vi "ColorArray2Ramp.vi"(11 "Color Array":u32[](array[colorbox])=[0, 16448250, 0]) -> (3 "Color Ramp (zero is black)":u32[](array[colorbox]))   [LabVIEW 2023]
panel:
  # "Overview: This These VI demonstrate algorithms to generate color tables for LabVIEW color ramps.\nRequirements: LabVIEW 2012\nInstructions:\n1. Set colors in color array\n2. Run VI\n3. Change speed\n4. try another colors combination"
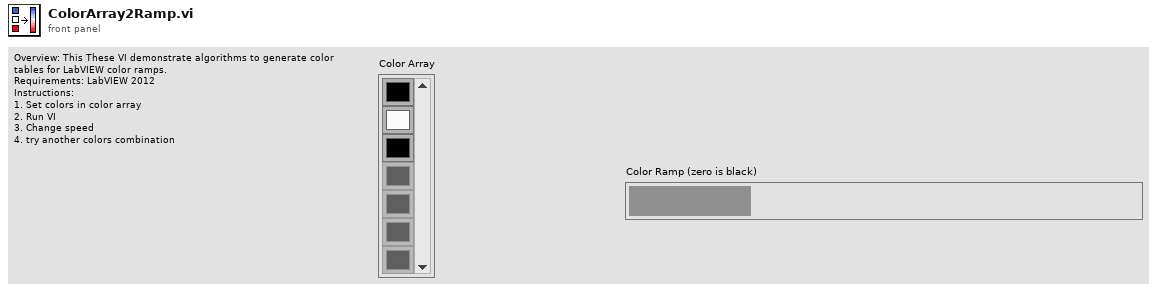
[diagram p1: front panel]
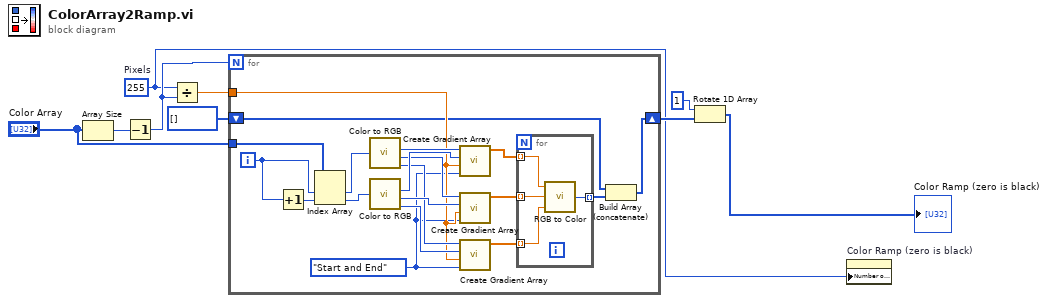
[diagram p0: block diagram]
diagram:
  w1 = 255  # Pixels
  n1 = Array Size(array="Color Array") -> (size(s)=w5:i32)
  n2 = Decrement(x=w5) -> (x-1=w6:i32)
  n3 = Divide(x=w1, y=w6) -> (x/y=w3:dbl)
  n4 = for {
    N: w6 -> [_]
    tunnel: "Color Array" -> [w28]
    tunnel: w3 -> [w17]
    shift-right: [w10] -> w8
    shift-left: u32[] [] -> [w11]
    i -> [w27]
    w16 = enum16{"Start", "End", "Start and End", "None"}."Start and End" ("Values to Include")
    n5 = Increment(x=w27) -> (x+1=w26:i32)
    n6 = Index Array(array=w28, index #1=w27, index #2=w26) -> (element #1=w25:u32, element #2=w24:u32)
    n7 = call <vilib>:"Color to RGB.vi"("Color"=w25) -> ("R"=w23:u8, "G"=w21:u8, "B"=w19:u8)  [unwired: 1 out]
    n8 = call <vilib>:"Color to RGB.vi"("Color"=w24) -> ("R"=w22:u8, "G"=w20:u8, "B"=w18:u8)  [unwired: 1 out]
    n9 = call "Create Gradient Array.vi"("Values to Include"=w16, "Array Length"=w17, "End Value"=w22, "Start Value"=w23) -> ("Output Array"=w15:dbl[])  [unwired: 7 in]
    n10 = call "Create Gradient Array.vi"("Values to Include"=w16, "Array Length"=w17, "End Value"=w20, "Start Value"=w21) -> ("Output Array"=w14:dbl[])  [unwired: 7 in]
    n11 = call "Create Gradient Array.vi"("Values to Include"=w16, "Array Length"=w17, "End Value"=w18, "Start Value"=w19) -> ("Output Array"=w13:dbl[])  [unwired: 7 in]
    n12 = for {
      tunnel: w15 -> [w31] mode=indexing
      tunnel: w14 -> [w32] mode=indexing
      tunnel: w13 -> [w30] mode=indexing
      tunnel: [w29] -> w12 mode=indexing
      n13 = call <vilib>:"RGB to Color.vi"("B"=w30, "G"=w32, "R"=w31) -> ("Color"=w29:u32)
    }
    n14 = Build Array (concatenate)(w11, w12) -> (w10:u32[])
  }
  n15 = Rotate 1D Array(1:w8, 2:1 ("n")) -> (0:→"Color Ramp (zero is black)":u32[])
  n16 = property on="Color Ramp (zero is black)" class="Tabl (strict)"("Number of Columns"=w1) -> ()  [unwired: 2 in, 2 out]
